vi "Clear System Error.vi"(8 "error in (no error)":errorcluster {"code" format="%.0x"}, 10 "Error Code":u16 format="%04x", 11 "Device ID (0)":i32) -> (0 "error out":errorcluster {"code" format="%.0x"}, 3 "Device ID out":i32)   [LabVIEW 2020, in "KEYENCE LJ-X8000A.lvlib"]
doc: "This function clears the following system error: g0x0085: The connected head type is different than when previously started.h \nWhen all of the system errors that are occurring are successfully cleared, the controller will start measurements."
uses:
  KEYENCE LJ-X8000A.lvlib
panel:
  # "(c) 2019 KEYENCE CORPORATION.  ALL RIGHTS RESERVED."
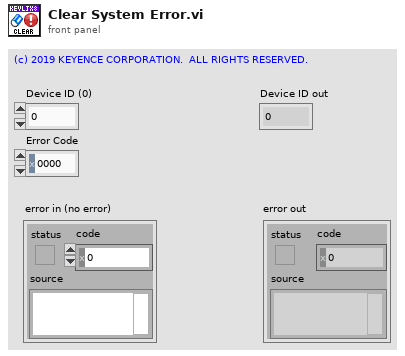
[diagram p1: front panel]
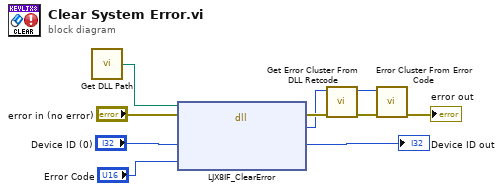
[diagram p0: block diagram]
diagram:
  n1 = call "Get DLL Path.vi"() -> ("DLL Path"=w7:path)  [unwired: 3 in]
  n2 = dll-call lib="C:/Program Files (x86)/National Instruments/LabVIEW 2018/instr.lib/KEYENCE LJ-X8000/LJX8_IF.*" fn="LJX8IF_ClearError"(path in=w7, error in="error in (no error)", "lDeviceId"="Device ID (0)", "wErrCode"="Error Code") -> (error out=w5:errorcluster, "lRetCode"=w4:i32, "lDeviceId"=→"Device ID out":i32)  [unwired: 2 in, 1 out]
  n3 = call "Get Error Cluster From DLL Retcode.vi"("error in (no error)"=w5, "DLL Return Code"=w4) -> ("error out"=w6:errorcluster, "VI Error Code"=w1:i32)  [unwired: 8 in]
  n4 = call <vilib>:"Error Cluster From Error Code.vi"("error in (no error)"=w6, "error code (0)"=w1) -> ("error out"=→"error out":errorcluster)  [unwired: 7 in]
